vi "Fishing OCR + Muti Area Capture.vi"() -> ()   [LabVIEW 2019]
doc: "This VI captures the region of the screen and displays it on the front panel continuously.\nCan be used to develop remote desktop applications."
uses:
  <vilib>/Utility/miscctls.llb/LVBoundsTypeDef.ctl
  System.Drawing
  <vilib>/Instr/_visa.llb/VISA Configure Serial Port (Instr).vi
  <vilib>/Utility/inputDevices.llb/mouseAcquire.vi
  <vilib>/Utility/inputDevices.llb/closeMouse.vi
  <vilib>/wsapi/NI_WebServices.lvlib
panel:
  out "TX":bool
  out "Scan Cycle":dbl
  out "Reset":bool
  out "Reset Var":bool
  out "Disable Timing":bool
  out "VISA":refnum<visa-resource-name>
  out "COM Status":bool
  in  "MC COM Port":refnum<visa-resource-name>="COM5"
  out "MLE Output":string
  out "Possible Inputs":string[](array[string])
  out "Input Likelihood":dbl[](array[numeric])
  out "Max Index":i32
  out "Write String":string
  in  "Manual Reset":bool
  in  "Timing Detected":bool
  out "Disable Space":bool
  out "Match Score":i32
  in  "Match Threshold":dbl=800.0
  out "Valid Range":bool
  in  "Error In 3":errorcluster
  in  "Space Detected":bool
  in  "Error In 2":errorcluster
  out "Post Processed Combo":picture
  in  "delay":u32=100
  in  "Error In":errorcluster
  out "Raw OCR Output":string
  in  "Combo y offset":i32=150
  in  "Combo x offset":i32=-100
  out "Combo":picture
  in  "Combo  Height  (px)":i32=50
  in  "Combo Width (px)":i32=360
  in  "Bar y offset":i32=200
  in  "Bar x offset":i32=-70
  out "Bar":picture
  in  "Bar Height  (px)":i32=30
  in  "Bar Width (px)":i32=280
  in  "Space Height (px)":i32=60
  in  "Space Width (px)":i32=145
  out "Space":picture
  in  "stop":bool
  # "Controls, Parameters, and Debug"
  # "Space Initiation"
  # "Bar Timing"
  # "Combo OCR"
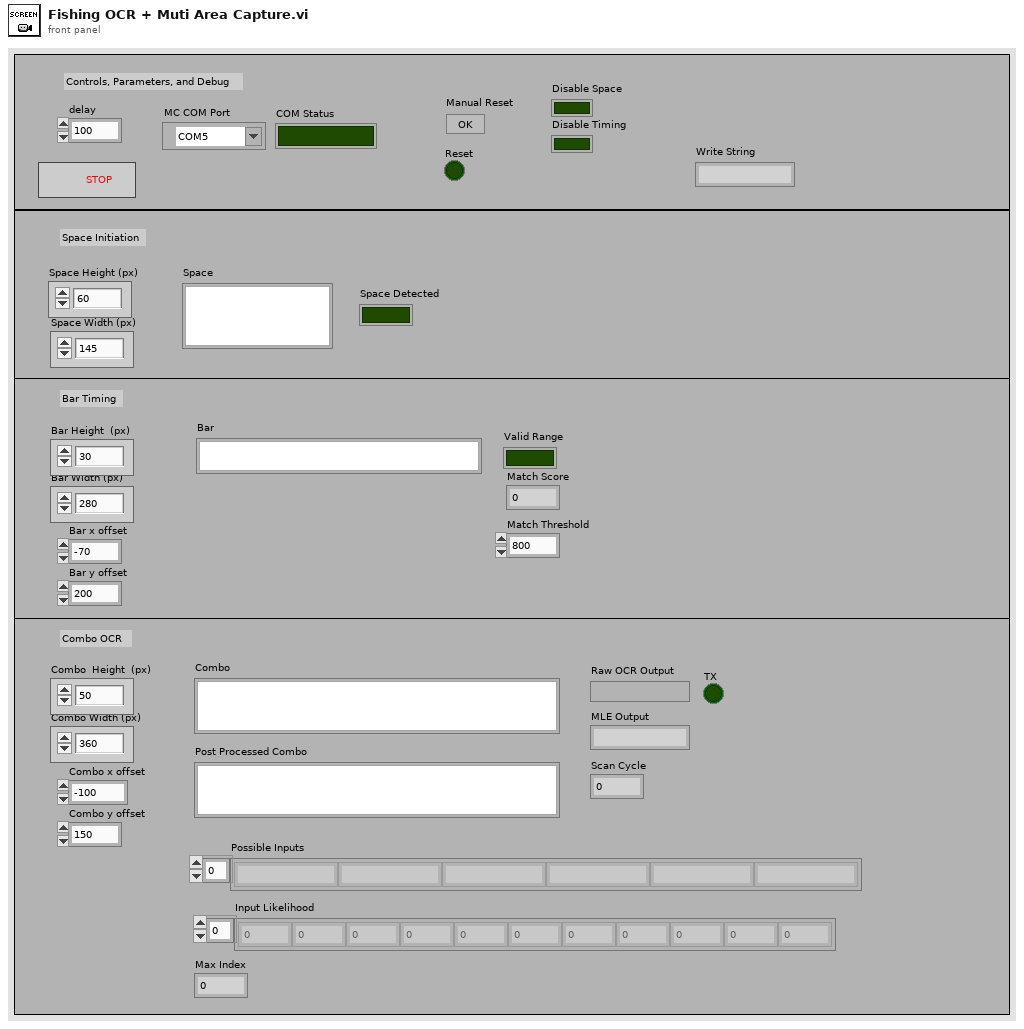
[diagram p1: front panel]
types:
  T1 = typedef "LVBoundsTypeDef.ctl" = cluster{"Width":u32, "Height":u32}
  T2 = typedef "Image Type" = u32
  T3 = cluster{"Horizontal":i32, "Vertical":i32, "Scrolling":i32}
  T4 = typedef "IMAQ Image.ctl" = refnum<image>
  T5 = typedef "imagedata.ctl" = cluster{"image type":i32, "image depth":i32, "image":u8[], "mask":u8[], "colors":u32[], "Rectangle":cluster{"left":i16, "top":i16, "right":i16, "bottom":i16}}
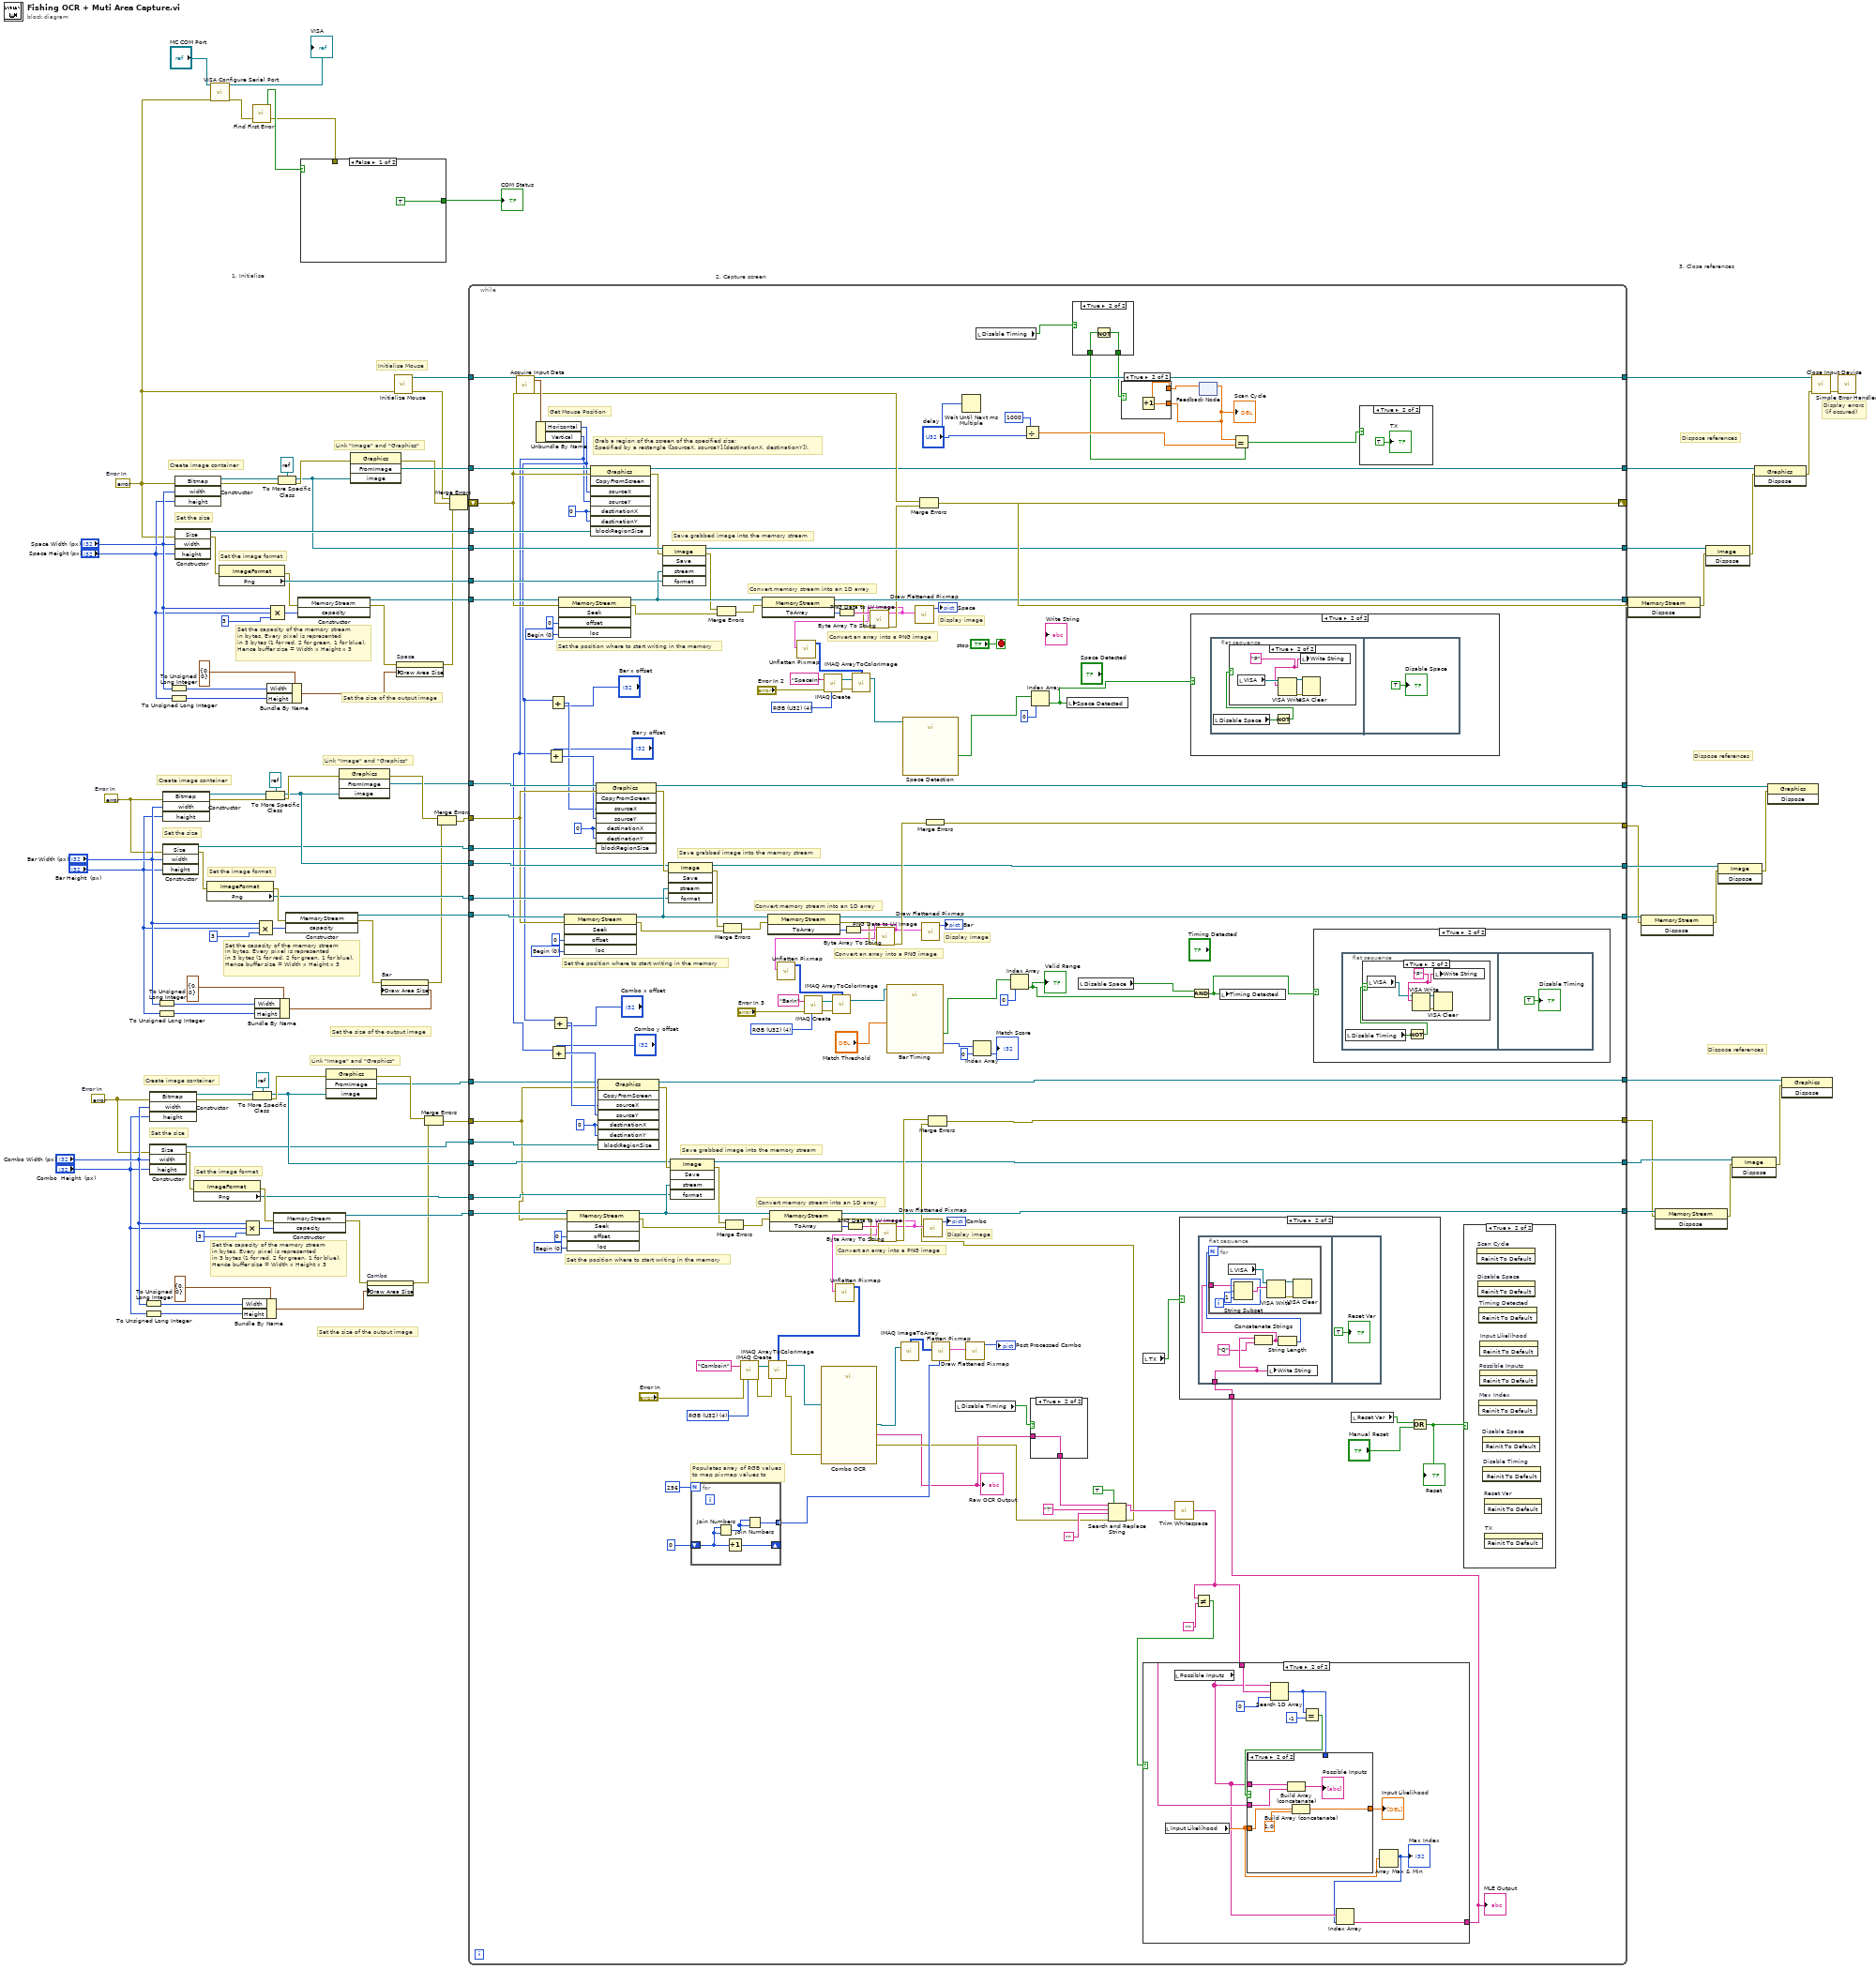
[diagram p0: block diagram]
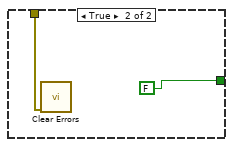
[diagram p2: hidden frame]
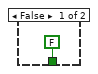
[diagram p4: hidden frame]
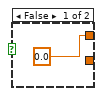
[diagram p5: hidden frame]
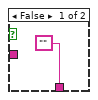
[diagram p11: hidden frame]
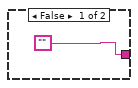
[diagram p12: hidden frame]
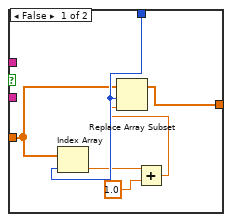
[diagram p13: hidden frame]
diagram:
  w23 = errorcluster {"status"=FALSE, "code"=0, "source"=""}  # Error In
  w53 = errorcluster {"status"=FALSE, "code"=0, "source"=""}  # Error In
  w2 = errorcluster {"status"=FALSE, "code"=0, "source"=""}  # Error In
  # "Dispose references"
  # "Link \"Image\" and \"Graphics\""
  # "Set the size"
  # "Create image container"
  # "Set the image format"
  # "Set the size of the output image"
  # "Set the capacity of the memory stream\nin bytes. Every pixel is represented\nin 3 bytes (1 for red, 2 for green, 1 for blue).\nHence buffer size = Width x Height x 3"
  # "Dispose references"
  # "Link \"Image\" and \"Graphics\""
  # "Set the size"
  # "Create image container"
  # "Set the image format"
  # "Set the size of the output image"
  # "Set the capacity of the memory stream\nin bytes. Every pixel is represented\nin 3 bytes (1 for red, 2 for green, 1 for blue).\nHence buffer size = Width x Height x 3"
  # "Link \"Image\" and \"Graphics\""
  # "Set the size"
  # "Create image container"
  # "3. Close references"
  # "2. Capture screen"
  # "1. Initialise"
  # "Display errors\n (if occured)"
  # "Dispose references"
  # "Set the image format"
  # "Set the size of the output image"
  # "Set the capacity of the memory stream\nin bytes. Every pixel is represented\nin 3 bytes (1 for red, 2 for green, 1 for blue).\nHence buffer size = Width x Height x 3"
  # "Initialise Mouse"
  n1 = To Unsigned Long Integer(number="Combo Width (px)") -> (unsigned 32bit integer=w26:u32)
  n2 = To Unsigned Long Integer(number="Combo  Height  (px)") -> (unsigned 32bit integer=w24:u32)
  n3 = constructor class="Bitmap"(error in=w23, "width"="Combo Width (px)", "height"="Combo  Height  (px)") -> (reference out=w34:refnum<k24>, error out=w36:errorcluster)  [unwired: 2 in, 3 out]
  n4 = constructor class="Size"(error in=w23, "width"="Combo Width (px)", "height"="Combo  Height  (px)") -> (reference out=w19:refnum<k24>, error out=w30:errorcluster)  [unwired: 2 in, 3 out]
  n5 = To Unsigned Long Integer(number="Bar Width (px)") -> (unsigned 32bit integer=w56:u32)
  n6 = To Unsigned Long Integer(number="Bar Height  (px)") -> (unsigned 32bit integer=w54:u32)
  n7 = constructor class="Bitmap"(error in=w53, "width"="Bar Width (px)", "height"="Bar Height  (px)") -> (reference out=w64:refnum<k24>, error out=w66:errorcluster)  [unwired: 2 in, 3 out]
  n8 = constructor class="Size"(error in=w53, "width"="Bar Width (px)", "height"="Bar Height  (px)") -> (reference out=w49:refnum<k24>, error out=w60:errorcluster)  [unwired: 2 in, 3 out]
  n9 = To Unsigned Long Integer(number="Space Width (px)") -> (unsigned 32bit integer=w75:u32)
  n10 = To Unsigned Long Integer(number="Space Height (px)") -> (unsigned 32bit integer=w73:u32)
  n11 = constructor class="Bitmap"(error in=w2, "width"="Space Width (px)", "height"="Space Height (px)") -> (reference out=w95:refnum<k24>, error out=w98:errorcluster)  [unwired: 2 in, 3 out]
  n12 = constructor class="Size"(error in=w2, "width"="Space Width (px)", "height"="Space Height (px)") -> (reference out=w93:refnum<k24>, error out=w84:errorcluster)  [unwired: 2 in, 3 out]
  n13 = property class="ImageFormat"(error in=w30) -> (error out=w29:errorcluster, "Png"=w21:refnum<k24>)  [unwired: 1 in, 1 out]
  n14 = property class="ImageFormat"(error in=w60) -> (error out=w59:errorcluster, "Png"=w51:refnum<k24>)  [unwired: 1 in, 1 out]
  n15 = call-poly "VISA Configure Serial Port"("VISA resource name"="MC COM Port", "error in (no error)"=w2) -> ("VISA resource name out"=→"VISA":refnum<visa-resource-name>, "error out"=w7:errorcluster)  [unwired: 12 in]
  n16 = property class="ImageFormat"(error in=w84) -> (error out=w83:errorcluster, "Png"=w92:refnum<k24>)  [unwired: 1 in, 1 out]
  n17 = Bundle By Name(cluster=T1 {"Width"=0, "Height"=0} ("Draw Area Size"), "Width"=w26, "Height"=w24) -> (w10:T1)
  n18 = Compound Arithmetic op=MULTIPLY("Combo Width (px)", "Combo  Height  (px)", 3 ("value")) -> (w32:i32)
  n19 = call <vilib>:"Find First Error.vi"("error in (no error)"=w7) -> ("error out"=w4:errorcluster, "error?"=w6:bool)  [unwired: 3 in]
  n20 = To More Specific Class(target class=refnum<k24> refnum, reference=w34, error in=w36) -> (specific class reference=w20:refnum<k24>, error out=w37:errorcluster)
  n21 = Bundle By Name(cluster=T1 {"Width"=0, "Height"=0} ("Draw Area Size"), "Width"=w56, "Height"=w54) -> (w38:T1)
  n22 = Compound Arithmetic op=MULTIPLY("Bar Width (px)", "Bar Height  (px)", 3 ("value")) -> (w62:i32)
  n23 = To More Specific Class(target class=refnum<k24> refnum, reference=w64, error in=w66) -> (specific class reference=w50:refnum<k24>, error out=w67:errorcluster)
  n24 = Bundle By Name(cluster=T1 {"Width"=0, "Height"=0} ("Draw Area Size"), "Width"=w75, "Height"=w73) -> (w79:T1)
  n25 = Compound Arithmetic op=MULTIPLY("Space Width (px)", "Space Height (px)", 3 ("value")) -> (w87:i32)
  n26 = constructor class="MemoryStream"(error in=w29, "capacity"=w32) -> (reference out=w22:refnum<k24>, error out=w9:errorcluster)  [unwired: 2 in, 2 out]
  n27 = To More Specific Class(target class=refnum<k24> refnum, reference=w95, error in=w98) -> (specific class reference=w86:refnum<k24>, error out=w99:errorcluster)
  n28 = constructor class="MemoryStream"(error in=w59, "capacity"=w62) -> (reference out=w52:refnum<k24>, error out=w39:errorcluster)  [unwired: 2 in, 2 out]
  n29 = constructor class="MemoryStream"(error in=w83, "capacity"=w87) -> (reference out=w89:refnum<k24>, error out=w78:errorcluster)  [unwired: 2 in, 2 out]
  n30 = case shown="False" w6 {
    tunnel: [TRUE FALSE] -> w5
    tunnel: w4 -> [_ w103]
    frame False {
    }
    frame True {
      n31 = call <vilib>:"Clear Errors.vi"("error in (no error)"=w103) -> ()  [unwired: 5 in, 2 out]
    }
  }
  "COM Status" <- w5
  n32 = invoke class="Graphics" method="FromImage"(error in=w37, "image"=w20) -> (error out=w28:errorcluster, "FromImage"=w18:refnum<k24>)  [unwired: 2 in, 2 out]
  n33 = invoke class="Graphics" method="FromImage"(error in=w67, "image"=w50) -> (error out=w58:errorcluster, "FromImage"=w48:refnum<k24>)  [unwired: 2 in, 2 out]
  n34 = invoke class="Graphics" method="FromImage"(error in=w99, "image"=w86) -> (error out=w82:errorcluster, "FromImage"=w96:refnum<k24>)  [unwired: 2 in, 2 out]
  n35 = property on="Combo" class="Pict"(error in=w9, "Draw Area Size"=w10) -> (error out=w8:errorcluster)  [unwired: 1 in, 1 out]
  n36 = property on="Bar" class="Pict"(error in=w39, "Draw Area Size"=w38) -> (error out=w40:errorcluster)  [unwired: 1 in, 1 out]
  n37 = call <vilib>:"Initialize Mouse.vi"("error in (no error)"=w2) -> ("error out"=w80:errorcluster, "device ID"=w101:refnum<k1>)  [unwired: 9 in]
  n38 = property on="Space" class="Pict"(error in=w78, "Draw Area Size"=w79) -> (error out=w77:errorcluster)  [unwired: 1 in, 1 out]
  n39 = Merge Errors(w28, w8) -> (w17:errorcluster)
  n40 = Merge Errors(w58, w40) -> (w47:errorcluster)
  n41 = Merge Errors(w80, w82, w77) -> (w81:errorcluster)
  n42 = while {
    tunnel: w101 -> [w257]
    tunnel: [w255] -> w100
    tunnel: w96 -> [w254]
    tunnel: [w251] -> w94
    tunnel: w93 -> [w250]
    tunnel: w92 -> [w249]
    tunnel: [w248] -> w91
    tunnel: w89 -> [w247]
    tunnel: w86 -> [w240]
    shift-right: [w231] -> w72
    shift-left: w81 -> [w234]
    tunnel: [w230] -> w71
    tunnel: w52 -> [w216]
    tunnel: w51 -> [w215]
    tunnel: w50 -> [w214]
    tunnel: w49 -> [w213]
    tunnel: w48 -> [w212]
    tunnel: w47 -> [w211]
    tunnel: [w210] -> w44
    tunnel: [w209] -> w43
    tunnel: [w208] -> w42
    tunnel: [w207] -> w41
    tunnel: w22 -> [w185]
    tunnel: w21 -> [w184]
    tunnel: w20 -> [w183]
    tunnel: w19 -> [w182]
    tunnel: w18 -> [w181]
    tunnel: w17 -> [w180]
    tunnel: [w177] -> w14
    tunnel: [w176] -> w13
    tunnel: [w175] -> w12
    tunnel: [w174] -> w11
    stop <- "stop" stop-if-true
    w147 = T2 4 items=["Grayscale (U8)", "Grayscale (I16)", "Grayscale (SGL)", "Complex (CSG)", "RGB (U32)", "HSL (U32)", "RGB (U64)", "Grayscale (U16)"] ("Image Type")
    w158 = T2 4 items=["Grayscale (U8)", "Grayscale (I16)", "Grayscale (SGL)", "Complex (CSG)", "RGB (U32)", "HSL (U32)", "RGB (U64)", "Grayscale (U16)"] ("Image Type")
    w173 = T2 4 items=["Grayscale (U8)", "Grayscale (I16)", "Grayscale (SGL)", "Complex (CSG)", "RGB (U32)", "HSL (U32)", "RGB (U64)", "Grayscale (U16)"] ("Image Type")
    w196 = 0 ("destinationX")
    w199 = 0 items=["Begin", "Current", "End"] ("loc")
    w223 = 0 ("destinationX")
    w226 = 0 items=["Begin", "Current", "End"] ("loc")
    w241 = 0 ("destinationX")
    w245 = 0 items=["Begin", "Current", "End"] ("loc")
    # "Populates array of RGB values\nto map pixmap values to"
    # "Display image"
    # "Convert an array into a PNG image"
    # "Set the position where to start writing in the memory"
    # "Convert memory stream into an 1D array"
    # "Save grabbed image into the memory stream"
    # "Display image"
    # "Convert an array into a PNG image"
    # "Set the position where to start writing in the memory"
    # "Convert memory stream into an 1D array"
    # "Save grabbed image into the memory stream"
    # "Display image"
    # "Convert an array into a PNG image"
    # "Set the position where to start writing in the memory"
    # "Convert memory stream into an 1D array"
    # "Save grabbed image into the memory stream"
    # "Grab a region of the screen of the specified size;\nSpecified by a rectangle ([sourceX, sourceY],[destinationX, destinationY])."
    # "Get Mouse Position"
    n43 = call-poly <vilib>:"Acquire Input Data.vi"("device ID"=w257, "error in (no error)"=w234) -> ("device ID"=w255:refnum<k1>, "axis info"=w256:T3, "error out"=w233:errorcluster)  [unwired: 14 in, 1 out]
    n44 = Unbundle By Name(w256) -> ("Horizontal"=w179:i32, "Vertical"=w178:i32)
    n45 = Add(x=w178, y="Bar y offset") -> (x+y=w206:i32)
    n46 = Add(x=w179, y="Bar x offset") -> (x+y=w205:i32)
    n47 = Add(x=w178, y="Combo y offset") -> (x+y=w189:i32)
    n48 = Add(x=w179, y="Combo x offset") -> (x+y=w188:i32)
    n49 = invoke class="MemoryStream" method="Seek"(reference=w247, error in=w234, "offset"=i64 0, "loc"=w245) -> (reference out=w242:refnum<k24>, error out=w237:errorcluster)  [unwired: 1 in, 3 out]
    n50 = invoke class="MemoryStream" method="Seek"(reference=w216, error in=w211, "offset"=i64 0, "loc"=w226) -> (reference out=w224:refnum<k24>, error out=w220:errorcluster)  [unwired: 1 in, 3 out]
    n51 = invoke class="MemoryStream" method="Seek"(reference=w185, error in=w180, "offset"=i64 0, "loc"=w199) -> (reference out=w197:refnum<k24>, error out=w193:errorcluster)  [unwired: 1 in, 3 out]
    n52 = invoke class="Graphics" method="CopyFromScreen"(reference=w254, error in=w234, "sourceX"=w179, "sourceY"=w178, "destinationX"=w241, "destinationY"=w241, "blockRegionSize"=w250) -> (reference out=w230:refnum<k24>, error out=w235:errorcluster)  [unwired: 1 in, 6 out]
    n53 = invoke class="Graphics" method="CopyFromScreen"(reference=w212, error in=w211, "sourceX"=w205, "sourceY"=w206, "destinationX"=w223, "destinationY"=w223, "blockRegionSize"=w213) -> (reference out=w209:refnum<k24>, error out=w218:errorcluster)  [unwired: 1 in, 6 out]
    n54 = invoke class="Graphics" method="CopyFromScreen"(reference=w181, error in=w180, "sourceX"=w188, "sourceY"=w189, "destinationX"=w196, "destinationY"=w196, "blockRegionSize"=w182) -> (reference out=w174:refnum<k24>, error out=w191:errorcluster)  [unwired: 1 in, 6 out]
    n55 = invoke class="Image" method="Save"(reference=w240, error in=w235, "stream"=w242, "format"=w249) -> (reference out=w248:refnum<k24>, error out=w238:errorcluster)  [unwired: 1 in, 3 out]
    n56 = invoke class="Image" method="Save"(reference=w214, error in=w218, "stream"=w224, "format"=w215) -> (reference out=w210:refnum<k24>, error out=w221:errorcluster)  [unwired: 1 in, 3 out]
    n57 = invoke class="Image" method="Save"(reference=w183, error in=w191, "stream"=w197, "format"=w184) -> (reference out=w176:refnum<k24>, error out=w194:errorcluster)  [unwired: 1 in, 3 out]
    n58 = for {
      N: 256 -> [_]
      tunnel: [w320] -> w159 mode=indexing
      shift-right: [w319] -> _
      shift-left: u8 0 -> [w317]
      n59 = Join Numbers(hi=w317, lo=w317) -> ((hi.lo)=w318:u16)
      n60 = Increment(x=w317) -> (x+1=w319:u8)
      n61 = Join Numbers(hi=w318, lo=w318) -> ((hi.lo)=w320:u32)
    }
    n62 = Merge Errors(w238, w237) -> (w236:errorcluster)
    n63 = Merge Errors(w221, w220) -> (w219:errorcluster)
    n64 = Merge Errors(w194, w193) -> (w192:errorcluster)
    n65 = call "IMAQ Create"("Image Name"="Comboin", "Image Type"=w173, "error in (no error)"="Error In") -> ("New Image"=w172:T4, "error out"=w171:errorcluster)  [unwired: 1 in, 1 out]
    n66 = invoke class="MemoryStream" method="ToArray"(reference=w242, error in=w236) -> (reference out=w251:refnum<k24>, error out=w239:errorcluster, "ToArray"=w253:u8[])  [unwired: 1 in]
    n67 = invoke class="MemoryStream" method="ToArray"(reference=w224, error in=w219) -> (reference out=w208:refnum<k24>, error out=w222:errorcluster, "ToArray"=w229:u8[])  [unwired: 1 in]
    n68 = invoke class="MemoryStream" method="ToArray"(reference=w197, error in=w192) -> (reference out=w177:refnum<k24>, error out=w195:errorcluster, "ToArray"=w202:u8[])  [unwired: 1 in]
    n69 = call "IMAQ Create"("Image Name"="BarIn", "Image Type"=w147, "error in (no error)"="Error In 3") -> ("New Image"=w146:T4, "error out"=w145:errorcluster)  [unwired: 1 in, 1 out]
    n70 = call "IMAQ Create"("Image Name"="SpaceIn", "Image Type"=w158, "error in (no error)"="Error In 2") -> ("New Image"=w157:T4, "error out"=w156:errorcluster)  [unwired: 1 in, 1 out]
    n71 = Byte Array To String(unsigned byte array=w253) -> (string=w252:string)
    n72 = Byte Array To String(unsigned byte array=w229) -> (string=w228:string)
    n73 = Byte Array To String(unsigned byte array=w202) -> (string=w201:string)
    n74 = call <vilib>:"PNG Data to LV Image.vi"("error in (no error)"=w239, "png data"=w252) -> ("error out"=w232:errorcluster, "image data"=w154:T5)  [unwired: 8 in]
    n75 = call <vilib>:"Unflatten Pixmap.vi"("image data"=w154) -> ("24-bit pixmap"=w153:u32[][])  [unwired: 4 in, 6 out]
    n76 = call "IMAQ ArrayToColorImage"("Image Pixels (U32)"=w153, "Image"=w157, "error in (no error)"=w156) -> ("Image Out"=w152:T4)  [unwired: 2 in, 1 out]
    n77 = call <vilib>:"PNG Data to LV Image.vi"("error in (no error)"=w222, "png data"=w228) -> ("error out"=w217:errorcluster, "image data"=w141:T5)  [unwired: 8 in]
    n78 = call <vilib>:"Unflatten Pixmap.vi"("image data"=w141) -> ("24-bit pixmap"=w140:u32[][])  [unwired: 4 in, 6 out]
    n79 = call "IMAQ ArrayToColorImage"("Image Pixels (U32)"=w140, "Image"=w146, "error in (no error)"=w145) -> ("Image Out"=w142:T4)  [unwired: 2 in, 1 out]
    n80 = call <vilib>:"PNG Data to LV Image.vi"("error in (no error)"=w195, "png data"=w201) -> ("error out"=w190:errorcluster, "image data"=w168:T5)  [unwired: 8 in]
    n81 = call <vilib>:"Unflatten Pixmap.vi"("image data"=w168) -> ("24-bit pixmap"=w167:u32[][])  [unwired: 4 in, 6 out]
    n82 = call "IMAQ ArrayToColorImage"("Image Pixels (U32)"=w167, "Image"=w172, "error in (no error)"=w171) -> ("Image Out"=w169:T4, "error out"=w170:errorcluster)  [unwired: 2 in]
    n83 = call "Combo OCR"("Image In"=w169, "error in"=w170) -> ("Image Out"=w165:T4, "String (OCR/OCV 2)"=w121:string, "error out"=w129:errorcluster)  [unwired: 23 in]
    "Raw OCR Output" <- w121
    n84 = call "Bar Timing"("Image In"=w142, "Minimum Match Score (Color Matching 1)"="Match Threshold") -> ("Match Flag (Color Matching 1)"=w138:bool[], "Match Score (Color Matching 1)"=w136:i32[])  [unwired: 22 in, 2 out]
    n85 = call "IMAQ ImageToArray"("Image"=w165) -> ("Image Pixels (U8)"=w162:u8[][])  [unwired: 3 in, 4 out]
    n86 = call "Space Detection"("Image In"=w152) -> ("Match Flag (Color Matching 1)"=w149:bool[])  [unwired: 23 in, 3 out]
    n87 = call <vilib>:"Draw Flattened Pixmap.vi"("image data"=w154) -> ("new picture"=→"Space":picture)  [unwired: 8 in]
    n88 = Merge Errors(w233, w232) -> (w231:errorcluster)
    n89 = call <vilib>:"Draw Flattened Pixmap.vi"("image data"=w141) -> ("new picture"=→"Bar":picture)  [unwired: 8 in]
    n90 = call <vilib>:"Draw Flattened Pixmap.vi"("image data"=w168) -> ("new picture"=→"Combo":picture)  [unwired: 8 in]
    n91 = Merge Errors(w217) -> (w207:errorcluster)
    n92 = call <vilib>:"Flatten Pixmap.vi"("colors"=w159, "8-bit pixmap"=w162) -> ("image data"=w163:T5)  [unwired: 9 in]
    n93 = local read "Disable Timing"() -> (w107:bool)
    n94 = Wait Until Next ms Multiple(millisecond multiple="delay") -> ()  [unwired: 1 out]
    n95 = call <vilib>:"Draw Flattened Pixmap.vi"("image data"=w163) -> ("new picture"=→"Post Processed Combo":picture)  [unwired: 8 in]
    n96 = Index Array(array=w136, index=0) -> (element=→"Match Score":i32)
    n97 = local read "Disable Timing"() -> (w108:bool)
    n98 = Index Array(array=w138, index=0) -> (element=w124:bool)
    "Valid Range" <- w124
    n99 = Divide(x=1000, y="delay") -> (x/y=w114:dbl)
    n100 = case shown="True" w107 {
      tunnel: ["" w293] -> w122
      tunnel: w121 -> [_ w293]
      frame False {
      }
      frame True {
      }
    }
    n101 = Index Array(array=w149, index=0) -> (element=w115:bool)
    n102 = local write "Space Detected"(w115) -> ()
    n103 = local read "Disable Space"() -> (w123:bool)
    n104 = Search and Replace String(replace all?=TRUE ("replace all? (F)"), input string=w122, search string="?", replace string="", error in=w129) -> (result string=w130:string, error out=w128:errorcluster)  [unwired: 3 in, 2 out]
    n105 = Merge Errors(w190, w128) -> (w175:errorcluster)
    n106 = local read "TX"() -> (w105:bool)
    n107 = call <vilib>:"Trim Whitespace.vi"("string"=w130) -> ("trimmed string"=w126:string)  [unwired: 1 in]
    n108 = case shown="True" w115 {
      frame False {
      }
      frame True {
        n109 = flat-sequence {
          frame #0 {
            n110 = local read "Disable Space"() -> (w266:bool)
            n111 = Not(x=w266) -> (.not. x?=w265:bool)
            n112 = case shown="True" w265 {
              frame False {
              }
              frame True {
                w269 = "P" ("Write String")
                n113 = local read "VISA"() -> (w270:refnum<visa-resource-name>)
                n114 = VISA Write(VISA resource name=w270, write buffer=w269) -> (VISA resource name out=w267:refnum<visa-resource-name>, error out=w268:errorcluster)  [unwired: 1 in, 1 out]
                n115 = local write "Write String"(w269) -> ()
                n116 = VISA Clear(VISA resource name=w267, error in (no error)=w268) -> ()  [unwired: 2 out]
              }
            }
          }
          frame #1 {
            "Disable Space" <- TRUE ("Enable Space")
          }
        }
      }
    }
    n117 = And(x=w123, y=w124) -> (x .and. y?=w116:bool)
    n118 = Not Equal?(x=w126, y="") -> (x != y?=w125:bool)
    n119 = case shown="True" w125 {
      tunnel: w126 -> [_ w299]
      tunnel: ["" w295] -> w120
      frame False {
      }
      frame True {
        n120 = local read "Input Likelihood"() -> (w298:dbl[])
        n121 = local read "Possible Inputs"() -> (w297:string[])
        n122 = Search 1D Array(1D array=w297, element=w299, start index (0)=0) -> (index of element=w301:i32)
        n123 = Equal?(x=w301, y=-1) -> (x = y?=w302:bool)
        n124 = case shown="True" w302 {
          tunnel: w297 -> [_ w316]
          tunnel: w299 -> [_ w315]
          tunnel: w301 -> [w310 _]
          tunnel: w298 -> [w306 w312]
          tunnel: [w305 w313] -> w300
          frame False {
            n125 = Index Array(array=w306, index=w310) -> (element=w308:dbl)
            n126 = Add(x=w308, y=1.0) -> (x+y=w307:dbl)
            n127 = Replace Array Subset(array=w306, new element=w307, index=w310) -> (w305:dbl[])
          }
          frame True {
            n128 = Build Array (concatenate)(w316, w315) -> (→"Possible Inputs":string[])
            n129 = Build Array (concatenate)(w312, 1.0 ("new element/subarray")) -> (w313:dbl[])
          }
        }
        "Input Likelihood" <- w300
        n130 = Array Max & Min(array=w298) -> (max index (indices)=w296:i32)  [unwired: 3 out]
        "Max Index" <- w296
        n131 = Index Array(array=w297, index=w296) -> (element=w295:string)
      }
    }
    "MLE Output" <- w120
    n132 = case shown="True" w105 {
      tunnel: w120 -> [_ w272]
      frame False {
      }
      frame True {
        n133 = flat-sequence {
          tunnel: w272 -> [w276]
          frame #0 {
            n134 = Concatenate Strings(w276, "Q" ("string")) -> (w273:string)
            n135 = local write "Write String"(w276) -> ()
            n136 = String Length(string=w273) -> (length=w274:i32)
            n137 = for {
              N: w274 -> [_]
              tunnel: w273 -> [w277]
              i -> [w278]
              n138 = local read "VISA"() -> (w283:refnum<visa-resource-name>)
              n139 = String Subset(string=w277, offset (0)=w278, length (rest)=1 ("length (rest)")) -> (substring=w280:string)
              n140 = VISA Write(VISA resource name=w283, write buffer=w280) -> (VISA resource name out=w281:refnum<visa-resource-name>, error out=w282:errorcluster)  [unwired: 1 in, 1 out]
              n141 = VISA Clear(VISA resource name=w281, error in (no error)=w282) -> ()  [unwired: 2 out]
            }
          }
          frame #1 {
            "Reset Var" <- TRUE ("Reset Var")
          }
        }
      }
    }
    n142 = feedback #1() -> (w113:dbl)  [unwired: 1 in]
    "Scan Cycle" <- w113
    n143 = local write "Timing Detected"(w116) -> ()
    n144 = Equal?(x=w113, y=w114) -> (x = y?=w106:bool)
    n145 = case shown="True" w108 {
      tunnel: [FALSE w261] -> w112
      tunnel: w106 -> [_ w260]
      frame False {
      }
      frame True {
        n146 = Not(x=w260) -> (.not. x?=w261:bool)
      }
    }
    n147 = case shown="True" w112 {
      tunnel: [0.0 w264] -> w110
      tunnel: w113 -> [_ w263]
      frame False {
      }
      frame True {
        n148 = Increment(x=w263) -> (x+1=w264:dbl)
      }
    }
    n149 = feedback-in #1(w110) -> ()
    n150 = case shown="True" w116 {
      frame False {
      }
      frame True {
        n151 = flat-sequence {
          frame #0 {
            n152 = local read "Disable Timing"() -> (w286:bool)
            n153 = Not(x=w286) -> (.not. x?=w285:bool)
            n154 = case shown="True" w285 {
              frame False {
              }
              frame True {
                w290 = "P" ("Write String")
                n155 = local read "VISA"() -> (w289:refnum<visa-resource-name>)
                n156 = VISA Write(VISA resource name=w289, write buffer=w290) -> (VISA resource name out=w288:refnum<visa-resource-name>, error out=w287:errorcluster)  [unwired: 1 in, 1 out]
                n157 = local write "Write String"(w290) -> ()
                n158 = VISA Clear(VISA resource name=w288, error in (no error)=w287) -> ()  [unwired: 2 out]
              }
            }
          }
          frame #1 {
            "Disable Timing" <- TRUE ("Enable Space")
          }
        }
      }
    }
    n159 = local read "Reset Var"() -> (w117:bool)
    n160 = case shown="True" w106 {
      frame False {
      }
      frame True {
        "TX" <- TRUE ("TX")
      }
    }
    n161 = Or(x=w117, y="Manual Reset") -> (x .or. y?=w119:bool)
    "Reset" <- w119
    n162 = case shown="True" w119 {
      frame False {
      }
      frame True {
        n163 = invoke on="Scan Cycle" class="DigNum (strict)" method="Reinit To Default"() -> ()  [unwired: 3 in, 3 out]
        n164 = invoke on="Disable Space" class="Bool (strict)" method="Reinit To Default"() -> ()  [unwired: 3 in, 3 out]
        n165 = invoke on="Timing Detected" class="Bool (strict)" method="Reinit To Default"() -> ()  [unwired: 3 in, 3 out]
        n166 = invoke on="Max Index" class="DigNum (strict)" method="Reinit To Default"() -> ()  [unwired: 3 in, 3 out]
        n167 = invoke on="Possible Inputs" class="Arr (strict)" method="Reinit To Default"() -> ()  [unwired: 3 in, 3 out]
        n168 = invoke on="Input Likelihood" class="Arr (strict)" method="Reinit To Default"() -> ()  [unwired: 3 in, 3 out]
        n169 = invoke on="Disable Space" class="Bool (strict)" method="Reinit To Default"() -> ()  [unwired: 3 in, 3 out]
        n170 = invoke on="Disable Timing" class="Bool (strict)" method="Reinit To Default"() -> ()  [unwired: 3 in, 3 out]
        n171 = invoke on="Reset Var" class="Bool (strict)" method="Reinit To Default"() -> ()  [unwired: 3 in, 3 out]
        n172 = invoke on="TX" class="Bool (strict)" method="Reinit To Default"() -> ()  [unwired: 3 in, 3 out]
      }
    }
  }
  n173 = invoke class="MemoryStream" method="Dispose"(reference=w94, error in=w72) -> (error out=w90:errorcluster)  [unwired: 1 in, 2 out]
  n174 = invoke class="MemoryStream" method="Dispose"(reference=w42, error in=w41) -> (error out=w46:errorcluster)  [unwired: 1 in, 2 out]
  n175 = invoke class="MemoryStream" method="Dispose"(reference=w14, error in=w12) -> (error out=w16:errorcluster)  [unwired: 1 in, 2 out]
  n176 = invoke class="Image" method="Dispose"(reference=w91, error in=w90) -> (error out=w70:errorcluster)  [unwired: 1 in, 2 out]
  n177 = invoke class="Image" method="Dispose"(reference=w44, error in=w46) -> (error out=w45:errorcluster)  [unwired: 1 in, 2 out]
  n178 = invoke class="Image" method="Dispose"(reference=w13, error in=w16) -> (error out=w15:errorcluster)  [unwired: 1 in, 2 out]
  n179 = invoke class="Graphics" method="Dispose"(reference=w71, error in=w70) -> (error out=w69:errorcluster)  [unwired: 1 in, 2 out]
  n180 = invoke class="Graphics" method="Dispose"(reference=w43, error in=w45) -> ()  [unwired: 1 in, 3 out]
  n181 = invoke class="Graphics" method="Dispose"(reference=w11, error in=w15) -> ()  [unwired: 1 in, 3 out]
  n182 = call-poly <vilib>:"Close Input Device.vi"("error in (no error)"=w69, "device ID"=w100) -> ("error out"=w68:errorcluster)  [unwired: 8 in]
  n183 = call <vilib>:"Simple Error Handler.vi"("error in (no error)"=w68) -> ()  [unwired: 4 in, 5 out]
